vi "DAQmx Create Channel (TEDS-AI-Temperature-Thermocouple).vi"(0 "task in":refnum<k21>, 1 "maximum value":dbl=100.0 format="%0.2f", 2 "minimum value":dbl format="%0.2f", 5 "physical channels":tag, 6 "cjc source":i32(ring)=10116 items=["Built-In"=10200, "Constant Value"=10116, "Channel"=10113], 7 "name to assign":string, 9 "units":i32(ring)=10143 items=["Deg C"=10143, "Deg F"=10144, "Kelvins"=10325, "Deg R"=10145, "From Custom Scale"=10065], 10 "cjc channel":refnum<k21>, 11 "error in":errorcluster, 14 "cjc value":dbl=25.0 format="%0.2f") -> (4 "task out":refnum<k21>, 15 "error out":errorcluster)   [LabVIEW 2020]
doc: "Creates channel(s) that use a thermocouple to measure temperature. You must configure the physical channel(s) with TEDS information to use this VI."
uses:
  nilvaiu.dll
panel:
  # "input limits"
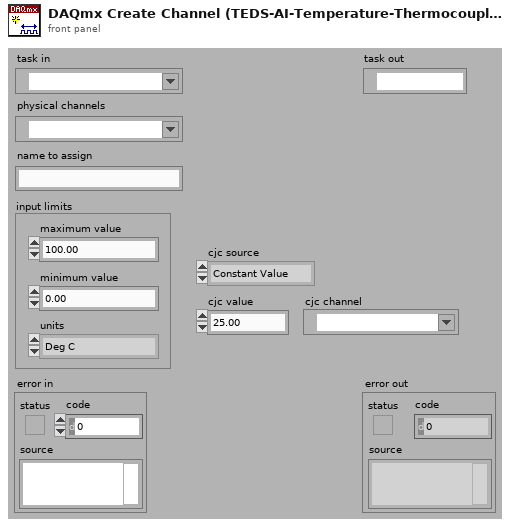
[diagram p1: front panel]
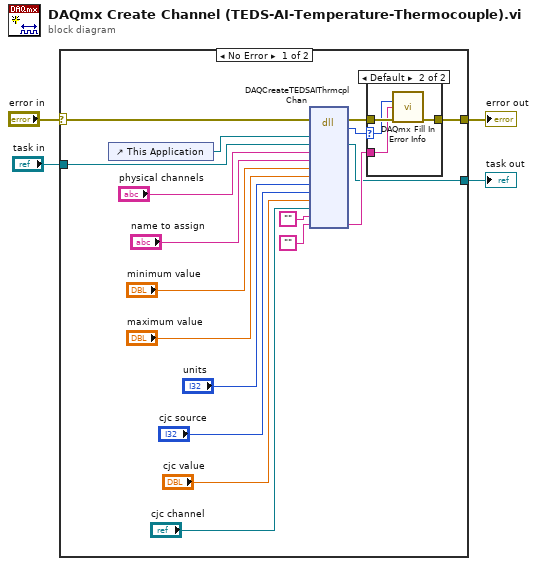
[diagram p0: block diagram]
diagram:
  n1 = case shown="No Error" "error in" {
    selector: "error in" -> [w8 w28]
    tunnel: "task in" -> [w10 w29]
    tunnel: [w9 w29] -> w3
    tunnel: [w7 w28] -> w1
    frame No Error {
      n2 = control-ref of="This Application"() -> (w16:refnum<vi>)
      n3 = dll-call lib="nilvaiu.*" fn="DAQCreateTEDSAIThrmcplChan"(error in=w8, "lvAppRef"=w16, "refObjPtr"=w10, "physicalChannelName"="physical channels", "channelNamesIn"="name to assign", "minVal"="minimum value", "maxVal"="maximum value", "units"="units", "cjcSource"="cjc source", "cjcVal"="cjc value", "cjcChannel"="cjc channel", "channelNamesOut"="", "extendedErrorInfo"="") -> (error out=w22:errorcluster, "return type"=w19:i32, "refObjPtr"=w9:refnum<k21>, "extendedErrorInfo"=w14:string)  [unwired: 12 in, 1 out]
      n4 = case shown="Default" w19 {
        selector: w19 -> [_ w25]
        tunnel: w22 -> [w23 w27]
        tunnel: [w23 w26] -> w7
        tunnel: w14 -> [_ w24]
        frame 0 {
        }
        frame Default {
          n5 = call "DAQmx Fill In Error Info.vi"("status code"=w25, "extended error info"=w24, "error in"=w27) -> ("error out"=w26:errorcluster)  [unwired: 1 in, 11 out]
        }
      }
    }
    frame Error {
    }
  }
  "task out" <- w3
  "error out" <- w1
